vi "CAN Read.vi"(8 "error in (no error)":errorcluster caption="错误输入（无错误）", 9 "TimestampBuffer":T1, 10 "MessageBuffer":T2, 11 "Channel":u8) -> (0 "error out":errorcluster caption="错误输出", 1 "TimestampBuffer out":T1, 2 "data":u8[](array[numeric]), 3 "function return":u32, 4 "ID":u32)   [LabVIEW 2021]
doc: "TPCANStatus __stdcall CAN_Read(\n TPCANHandle Channel, \n TPCANMsg* MessageBuffer, \n TPCANTimestamp* TimestampBuffer);"
uses:
  PCANBasic.dll
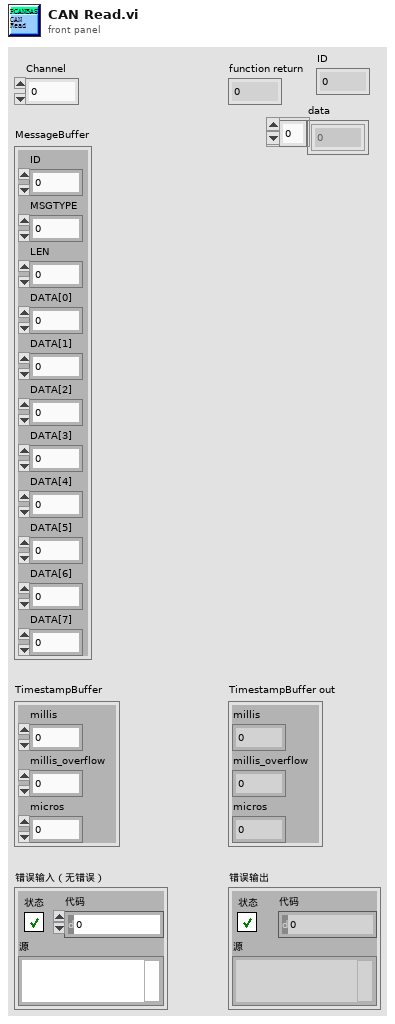
[diagram p1: front panel]
types:
  T1 = cluster{"millis":u32, "millis_overflow":u16, "micros":u16}
  T2 = cluster{"ID":u32, "MSGTYPE":u8, "LEN":u8, "DATA[0]":u8, "DATA[1]":u8, "DATA[2]":u8, "DATA[3]":u8, "DATA[4]":u8, "DATA[5]":u8, "DATA[6]":u8, "DATA[7]":u8}
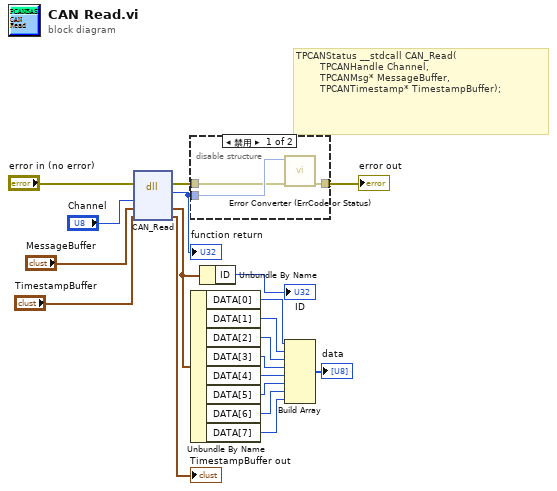
[diagram p0: block diagram]
diagram:
  # "TPCANStatus __stdcall CAN_Read(\n        TPCANHandle Channel, \n        TPCANMsg* MessageBuffer, \n        TPCANTimestamp* TimestampBuffer);"
  n1 = dll-call lib="D:/ON LINE WORK/LabVIEW/PCAN/PCAN 1.6(2021)/PCANBasic.*" fn="CAN_Read"(error in="error in (no error)", "Channel"="Channel", "MessageBuffer"="MessageBuffer", "TimestampBuffer"="TimestampBuffer") -> (error out=w13:errorcluster, "返回类型"=w19:u32, "MessageBuffer"=w2:T2, "TimestampBuffer"=→"TimestampBuffer out":T1)  [unwired: 3 in, 1 out]
  "function return" <- w19
  n2 = disable-structure shown="禁用" {
    disable-tunnel: w19 -> [w22 _]
    disable-tunnel: w13 -> [w21 _]
    disable-tunnel: [w20 _] -> w12
    frame Disabled {
      n3 = call "Error Converter (ErrCode or Status).vi"("error in (no error)"=w21, "error code"=w22) -> ("error out"=w20:errorcluster)  [unwired: 9 in]
    }
    frame Enabled {
    }
  }
  "error out" <- w12
  n4 = Unbundle By Name(w2) -> ("DATA[0]"=w11:u8, "DATA[1]"=w10:u8, "DATA[2]"=w9:u8, "DATA[3]"=w8:u8, "DATA[4]"=w7:u8, "DATA[5]"=w6:u8, "DATA[6]"=w5:u8, "DATA[7]"=w4:u8)
  n5 = Unbundle By Name(w2) -> ("ID"=→"ID":u32)
  n6 = Build Array(w11, w10, w9, w8, w7, w6, w5, w4) -> (→"data":u8[])
